vi "Progress bar.vi"(8 "error in":errorcluster, 10 "Current loop":i32, 11 "# loops":u8=18) -> (0 "error out":errorcluster, 3 "Progress":u8(slide) scale=0.0..18.0)   [LabVIEW 2024]
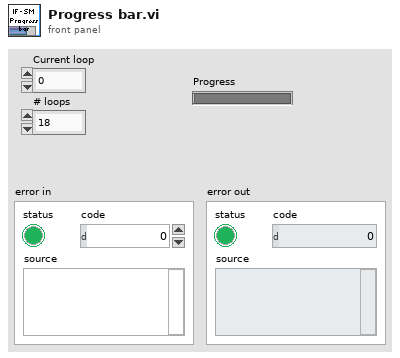
[diagram p1: front panel]
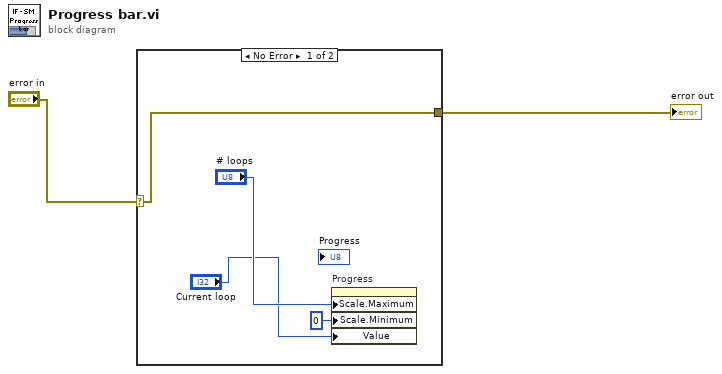
[diagram p0: block diagram]
diagram:
  n1 = case shown="No Error" "error in" {
    selector: "error in" -> [w6 w7]
    tunnel: [w6 w7] -> w1
    frame No Error {
      n2 = property on="Progress" class="Slide (strict)"("Scale.Maximum"="# loops", "Scale.Minimum"=u8 0 ("Scale.Range:Minimum"), "Value"="Current loop") -> ()  [unwired: 2 in, 2 out]
    }
    frame Error {
    }
  }
  "error out" <- w1
